vi "HP-disconnect.vi"(8 "error in (no error)":errorcluster, 11 "HP-S-Serial in":refnum<class "HP-S-Serial.lvclass">) -> (0 "error out":errorcluster, 3 "HP-S-Serial out":refnum<class "HP-S-Serial.lvclass">)   [LabVIEW 2020, in "HP-S-Serial.lvclass"]
uses:
  HP-S-Serial.lvclass
  HP-S-Serial.lvclass/HP-S-Serial.ctl
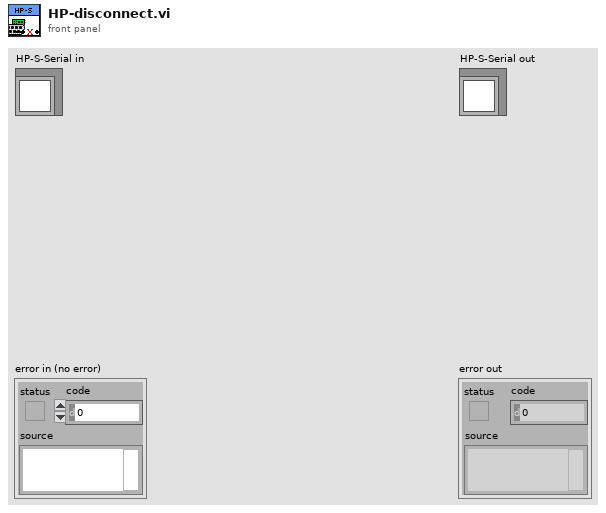
[diagram p1: front panel]
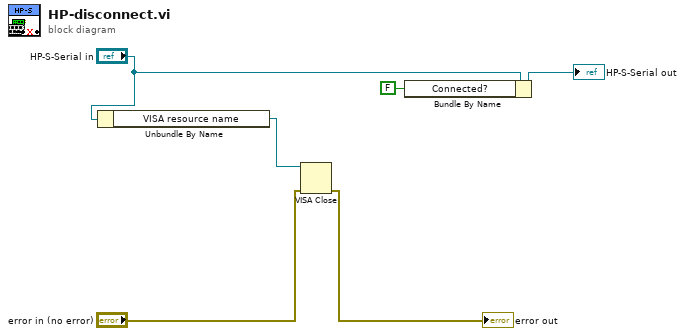
[diagram p0: block diagram]
diagram:
  n1 = Unbundle By Name("HP-S-Serial in") -> ("VISA resource name"=w5:refnum<visa-resource-name>)
  n2 = VISA Close(VISA resource name=w5, error in (no error)="error in (no error)") -> (error out=→"error out":errorcluster)
  n3 = Bundle By Name(cluster="HP-S-Serial in", "Connected?"=FALSE ("session.Connected?")) -> (→"HP-S-Serial out":refnum<class "HP-S-Serial.lvclass">)
